vi "7.2.-SubVI Entorno Virtual.vi"(6 "Axis label?":bool=TRUE, 7 "Radius":sgl=0.5, 9 "Character Size":sgl=10.0, 10 "COLOR EJE XYZ":u32(colorbox)=65295, 11 "Length":sgl=60.0) -> (3 "SceneObject out":refnum<vi>)   [LabVIEW 2020]
uses:
  <vilib>/picture/3D Picture Control/Object/Create Object (drawable).vi
  <vilib>/picture/3D Picture Control/Helpers/Apply Texture (no reference).vi
  <vilib>/picture/3D Picture Control/Object/Create Object (name).vi
  <vilib>/picture/3D Picture Control/NI_3D Picture Control.lvlib
panel:
  in  "COLOR OJO DER.":u32(colorbox)=65295
  in  "COLOR OJO IZQ.":u32(colorbox)=65295
  # "Visión Artificial - Realidad Virtual - Entorno Virtual\nDiego Cervantes Rodríguez\ndicer0.com"
  # "Programa que crea el entorno virtual 3D donde se mostrarán los objetos mostrados en las capturas"
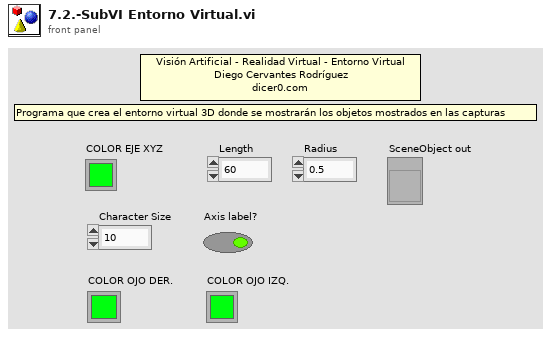
[diagram p1: front panel]
types:
  T1 = enum16{"No Filtration", "Linear Filtration", "Simple Mipmap Filtration", "Bilinear Filtration", "Trilinear Filtration"}
  T2 = typedef "imagedata.ctl" = cluster{"image type":i32, "image depth":i32, "image":u8[], "mask":u8[], "colors":u32[], "Rectangle":cluster{"left":i16, "top":i16, "right":i16, "bottom":i16}}
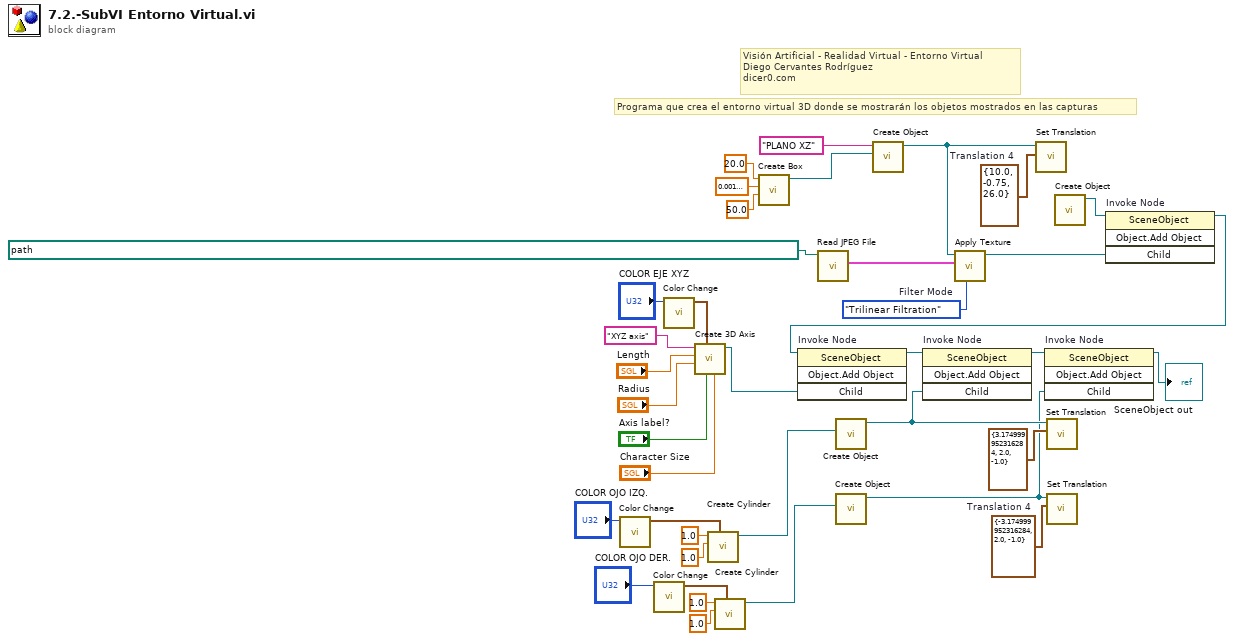
[diagram p0: block diagram]
diagram:
  w5 = cluster{"X":sgl, "Y":sgl, "Z":sgl} {"X"=-3.175, "Y"=2.0, "Z"=-1.0}  # Translation 4
  w38 = T1."Trilinear Filtration"  # Filter Mode
  w26 = cluster{"X":sgl, "Y":sgl, "Z":sgl} {"X"=10.0, "Y"=-0.75, "Z"=26.0}  # Translation 4
  # "Visión Artificial - Realidad Virtual - Entorno Virtual\nDiego Cervantes Rodríguez\ndicer0.com"
  # "Programa que crea el entorno virtual 3D donde se mostrarán los objetos mostrados en las capturas"
  n1 = call <vilib>:"Color Change.vi"("Color"="COLOR OJO IZQ.") -> ("RGBA"=w13:cluster{"R":sgl, "G":sgl, "B":sgl, "A":sgl})  [unwired: 10 in]
  n2 = call <vilib>:"Color Change.vi"("Color"="COLOR OJO DER.") -> ("RGBA"=w6:cluster{"R":sgl, "G":sgl, "B":sgl, "A":sgl})  [unwired: 10 in]
  n3 = call <vilib>:"Color Change.vi"("Color"="COLOR EJE XYZ") -> ("RGBA"=w34:cluster{"R":sgl, "G":sgl, "B":sgl, "A":sgl})  [unwired: 10 in]
  n4 = call <vilib>:"Create 3D Axis.vi"("Character Size"="Character Size", "Axis label?"="Axis label?", "Color"=w34, "Radius"="Radius", "Length"="Length", "Name"="XYZ axis") -> ("New Object Refnum"=w18:refnum<vi>)  [unwired: 4 in, 1 out]
  n5 = call <vilib>:"Create Cylinder.vi"("Color"=w13, "Radius"=sgl 1.0 ("Length Y 3"), "Height"=sgl 1.0 ("Length X 3")) -> ("New Cylinder Refnum"=w17:refnum<vi>)  [unwired: 7 in, 1 out]
  n6 = call <vilib>:"Create Cylinder.vi"("Color"=w6, "Radius"=sgl 1.0 ("Length Y 3"), "Height"=sgl 1.0 ("Length X 3")) -> ("New Cylinder Refnum"=w10:refnum<vi>)  [unwired: 7 in, 1 out]
  n7 = call <vilib>:"Create Box.vi"("Length Z"=sgl 50.0 ("Length Z 3"), "Length Y"=sgl 0.001 ("Length Y 3"), "Length X"=sgl 20.0 ("Length X 3")) -> ("New Box Refnum"=w25:refnum<vi>)  [unwired: 7 in, 1 out]
  n8 = call <vilib>:"Read JPEG File.vi"("path to JPEG file"=path "C:/Users/diego/OneDrive/Documents/Aprendiendo/LabVIEW/1.-Sistemas de Visión Artificial/Img/7.0.-Realidad Virtual - Estereoscopio/XZ_Grid.jpg") -> ("image data"=w36:T2)  [unwired: 8 in, 2 out]
  n9 = call-poly <vilib>:"Create Object.vi"("Geometry"=w17) -> ("Scene:New Object"=w11:refnum<vi>)  [unwired: 9 in, 1 out]
  n10 = call-poly <vilib>:"Create Object.vi"("Geometry"=w10) -> ("Scene:New Object"=w4:refnum<vi>)  [unwired: 9 in, 1 out]
  n11 = call-poly <vilib>:"Create Object.vi"("Geometry"=w25, "Name"="PLANO XZ") -> ("Scene:New Object"=w35:refnum<vi>)  [unwired: 8 in, 1 out]
  n12 = call-poly <vilib>:"Apply Texture.vi"("Filter Mode"=w38, "Image Data"=w36, "Scene Object In"=w35) -> ("Scene Object Out"=w19:refnum<vi>)  [unwired: 7 in, 1 out]
  n13 = call <vilib>:"Set Translation.vi"("Translation"=w26, "Scene Object"=w35) -> ()  [unwired: 8 in, 2 out]
  n14 = call <vilib>:"Set Translation.vi"("Translation"=cluster{"X":sgl, "Y":sgl, "Z":sgl} {"X"=3.175, "Y"=2.0, "Z"=-1.0} ("Translation 4"), "Scene Object"=w11) -> ()  [unwired: 8 in, 2 out]
  n15 = call <vilib>:"Set Translation.vi"("Translation"=w5, "Scene Object"=w4) -> ()  [unwired: 8 in, 2 out]
  n16 = call-poly <vilib>:"Create Object.vi"() -> ("Scene:New Object"=w20:refnum<vi>)  [unwired: 10 in, 1 out]
  n17 = invoke on="Invoke Node" class="SceneObject" method="Object.Add Object"(reference=w20, "Child"=w19) -> (reference out=w21:refnum<vi>)  [unwired: 2 in, 3 out]
  n18 = invoke on="Invoke Node" class="SceneObject" method="Object.Add Object"(reference=w21, "Child"=w18) -> (reference out=w3:refnum<vi>)  [unwired: 2 in, 3 out]
  n19 = invoke on="Invoke Node" class="SceneObject" method="Object.Add Object"(reference=w3, "Child"=w11) -> (reference out=w2:refnum<vi>)  [unwired: 2 in, 3 out]
  n20 = invoke on="Invoke Node" class="SceneObject" method="Object.Add Object"(reference=w2, "Child"=w4) -> (reference out=→"SceneObject out":refnum<vi>)  [unwired: 2 in, 3 out]
